vi "DIPinSelected.vi"(8 "错误输入（无错误）":errorcluster) -> (0 "错误输出":errorcluster)   [LabVIEW 2014]
uses:
  X86Dll/ZXUTConfigMgr.dll
panel:
  in  "管脚序号0~7":u8
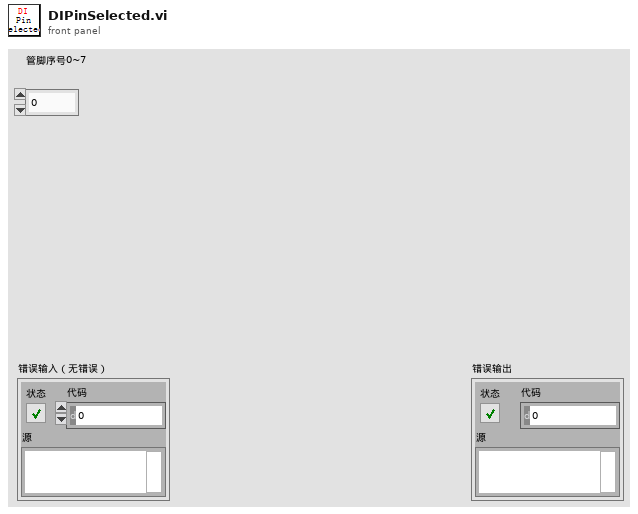
[diagram p1: front panel]
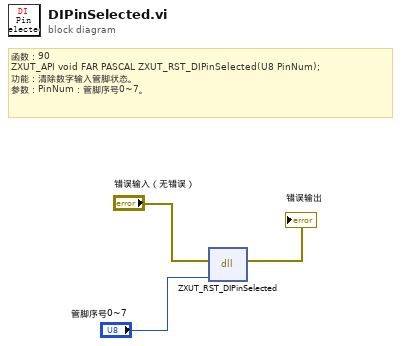
[diagram p0: block diagram]
diagram:
  # "函数：90\nZXUT_API void\tFAR PASCAL ZXUT_RST_DIPinSelected(U8 PinNum);\n功能：清除数字输入管脚状态。\n参数：PinNum：管脚序号0~7。"
  n1 = dll-call lib="D:/Software/Utrasonic on-line monitoring/X86Dll/ZXUTConfigMgr.dll" fn="ZXUT_RST_DIPinSelected"(error in="错误输入（无错误）", "PinNum"="管脚序号0~7") -> (error out=→"错误输出":errorcluster)  [unwired: 4 in, 1 out]
